vi "GetCalUnits.vi"(0 "Dynamic.lvclass":refnum<class "Dynamic.lvclass">) -> (6 "Calibration Units":string, 7 "dB On":bool)   [LabVIEW 2018, in "Measurement Channels.lvlib" / "Dynamic.lvclass"]
uses:
  Dynamic.lvclass
  SubVIs Table/Custom Ctls Table/ge_ColType.ctl
  Dynamic.lvclass/Dynamic.ctl
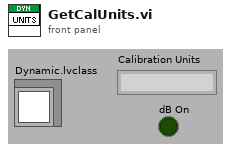
[diagram p1: front panel]
types:
  T1 = typedef "ge_ColType.ctl" = enum16{"Volts", "Amps", "Ohms", "TermCfg", "WireCfg", "Coup", "Slope", "Iex", "CalUnits", "ThrmUnits", "ThrmType", "CJCSrc", "BrdgType", "Strn Mode", "RTDType"}
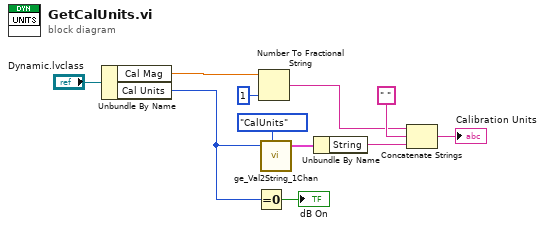
[diagram p0: block diagram]
diagram:
  n1 = Unbundle By Name("Dynamic.lvclass") -> ("Cal Mag"=w3:dbl, "Cal Units"=w2:u16)
  n2 = Equal To 0?(x=w2) -> (x = 0?=→"dB On":bool)
  n3 = Number To Fractional String(number=w3, precision (6)=i16 1) -> (F-format string=w5:string)  [unwired: 2 in]
  n4 = call "ge_Val2String_1Chan.vi"("Value"=w2, "ColType"=ge_ColType."CalUnits") -> ("String and Val"=w10:cluster{"String":string, "Value":u16})  [unwired: 5 in]
  n5 = Unbundle By Name(w10) -> ("String"=w9:string)
  n6 = Concatenate Strings(w5, " " ("string"), w9) -> (→"Calibration Units":string)
